vi "Add Timing Section.vi"(8 "error in":errorcluster, 11 "custom device in":T1 format="%.0x") -> (0 "error out":errorcluster, 2 "timing section":T1 format="%.0x", 3 "custom device out":T1 format="%.0x")   [LabVIEW 2020, in "Ballard MIL-STD-1553 Scripting.lvlib"]
uses:
  Ballard MIL-STD-1553 Scripting.lvlib
  <vilib>/NI VeriStand/Custom Device API/Custom Device Item Ref.ctl
  Constants.vi
  <vilib>/NI VeriStand/Custom Device API/Custom Device API.lvlib
  <vilib>/NI VeriStand/Custom Device API/Custom Device Channel Type.ctl
  <vilib>/NI VeriStand/Custom Device API/Custom Device Channel.ctl
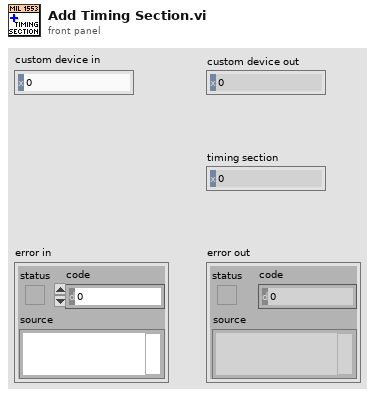
[diagram p1: front panel]
types:
  T1 = typedef "Custom Device API.lvlib/Custom Device Item Ref.ctl" = u64
  T2 = typedef "Custom Device API.lvlib/Custom Device Channel.ctl" = cluster{"Type":T3, "Units":string, "Default Value":dbl, "Faultable":bool, "Scalable":bool}
  T3 = typedef "Custom Device API.lvlib/Custom Device Channel Type.ctl" = enum16{"Input", "Output"}
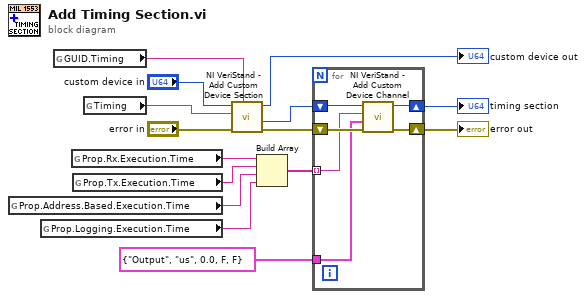
[diagram p0: block diagram]
diagram:
  n1 = global read "Constants.vi" "Prop.Address.Based.Execution.Time"() -> (w4:string)
  n2 = global read "Constants.vi" "Prop.Logging.Execution.Time"() -> (w3:string)
  n3 = global read "Constants.vi" "GUID.Timing"() -> (w12:string)
  n4 = global read "Constants.vi" "Prop.Rx.Execution.Time"() -> (w6:string)
  n5 = global read "Constants.vi" "Prop.Tx.Execution.Time"() -> (w5:string)
  n6 = global read "Constants.vi" "Timing"() -> (w11:string)
  n7 = call <vilib>:"NI VeriStand - Add Custom Device Section.vi"("GUID (Default Section)"=w12, "error in (no error)"="error in", "Section Name"=w11, "Parent Ref in"="custom device in") -> ("error out"=w10:errorcluster, "Section Ptr"=w9:T1, "Parent Ref out"=→"custom device out":T1)  [unwired: 4 in, 1 out]
  n8 = Build Array(w6, w5, w4, w3) -> (w2:string[])
  n9 = for {
    shift-right: [w19] -> w7
    shift-left: w10 -> [w21]
    shift-right: [w18] -> w8
    shift-left: w9 -> [w20]
    tunnel: w2 -> [w17] mode=indexing
    tunnel: T2 {"Type"=enum."Output", "Units"="us", "Default Value"=0.0, "Faultable"=FALSE, "Scalable"=FALSE} ("Channel") -> [w16]
    n10 = call <vilib>:"NI VeriStand - Add Custom Device Channel.vi"("error in (no error)"=w21, "Channel"=w16, "Channel Name"=w17, "Parent Ref in"=w20) -> ("error out"=w19:errorcluster, "Parent Ref out"=w18:T1)  [unwired: 4 in, 2 out]
  }
  "error out" <- w7
  "timing section" <- w8
